vi "equal.vi"(1 "Symbol Size":i32, 2 "Number of Subcarriers":i32, 3 "Channel Taps":cdb[](array[numeric]), 4 "Unequalized Signal":cdb[](array[numeric])) -> (0 "Equalized Signal":cdb[](array[numeric]))   [LabVIEW 2013]
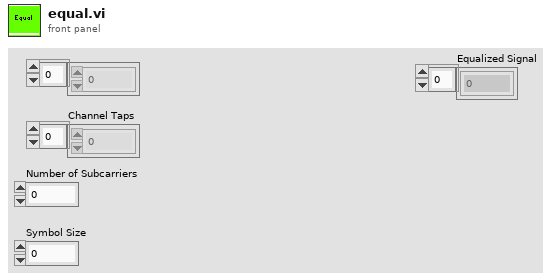
[diagram p1: front panel]
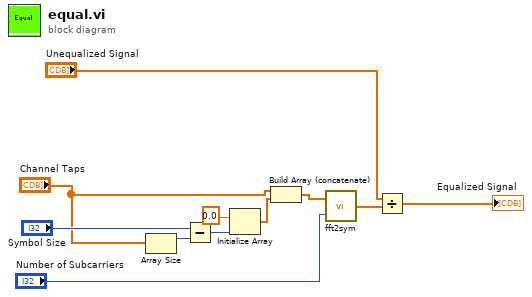
[diagram p0: block diagram]
diagram:
  n1 = Array Size(array="Channel Taps") -> (size(s)=w9:i32)
  n2 = Subtract(x="Symbol Size", y=w9) -> (x-y=w10:i32)
  n3 = Initialize Array(0.0 ("element"), w10) -> (w8:dbl[])
  n4 = Build Array (concatenate)("Channel Taps", w8) -> (w4:cdb[])
  n5 = call "fft2sym.vi"("Number of Subcarriers"="Number of Subcarriers", "Time domain In"=w4) -> ("Parallel Symbole out 2"=w3:cdb[])
  n6 = Divide(x="Unequalized Signal", y=w3) -> (x/y=→"Equalized Signal":cdb[])
